vi "Set Speed.vi"(8 "error in (no error)":errorcluster, 10 "Flow Rate (mL/min)":dbl format="%.2f", 11 "VICI Settings In":T1) -> (0 "error out":errorcluster, 1 "Connection Error":bool, 3 "VICI Settings Out":T1)   [LabVIEW 2018, in "VICI M6 M50 Party Mode.lvlib"]
uses:
  VICI M6 M50 Party Mode.lvlib
  Settings Cluster.ctl
  VICI Global Library.lvlib
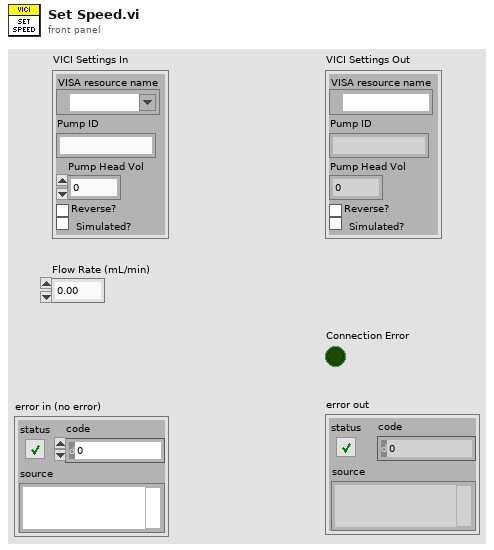
[diagram p1: front panel]
types:
  T1 = typedef "VICI M6 M50 Party Mode.lvlib/Settings Cluster.ctl" = cluster{"VISA resource name":refnum<visa-resource-name>, "Pump ID":string, "Pump Head Vol":dbl, "Reverse?":bool, "Simulated?":bool}
  T2 = typedef "VICI M6 M50 Party Mode.lvlib/VICI Global Library.lvlib/VICI Global.ctl" = cluster{"Busy":bool, "VISA #":string, "Current Pump":string, "Current Function":string, "Pump Array":string[], "Last Success":timestamp, "ID Queue":string[]}
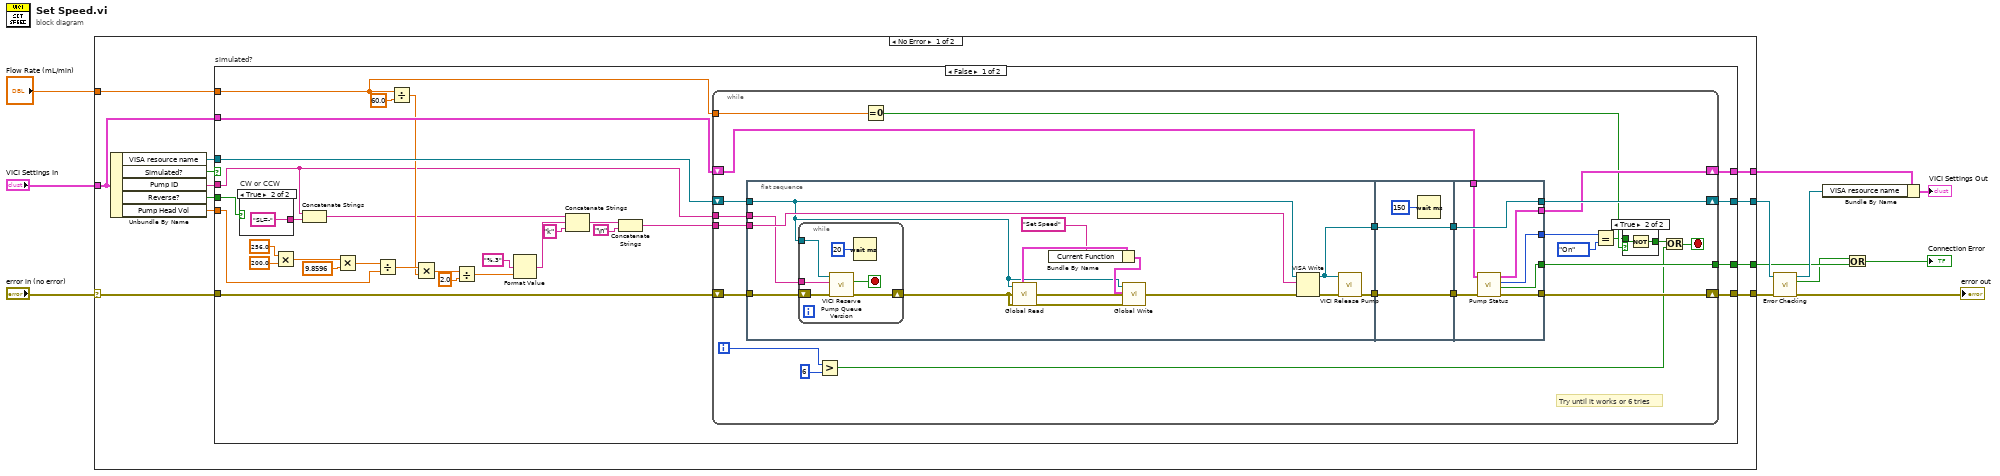
[diagram p0: block diagram]
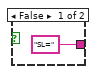
[diagram p3: hidden frame]
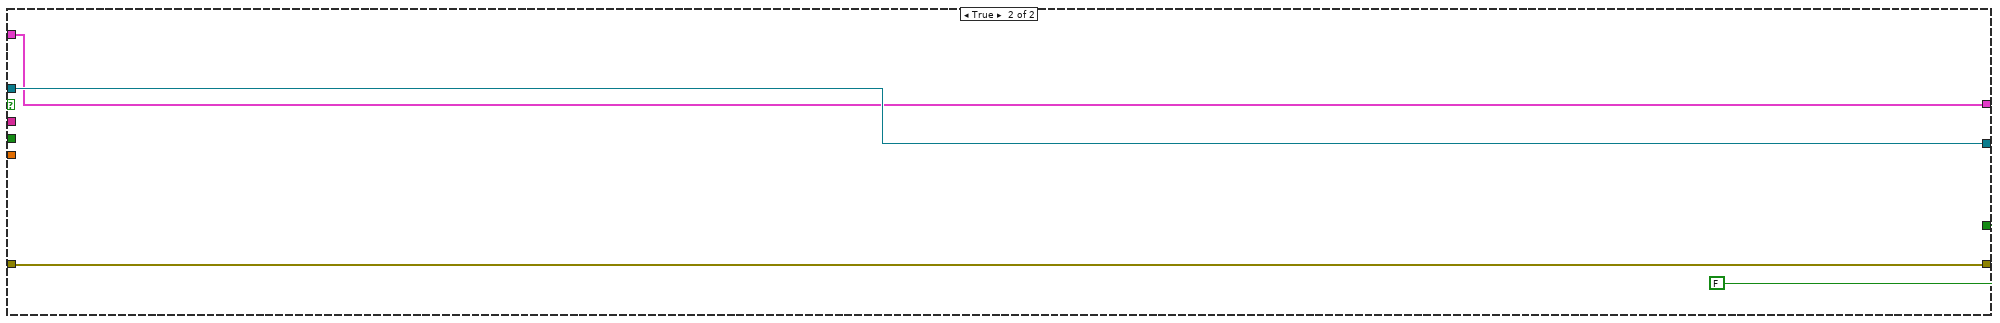
[diagram p4: hidden frame]
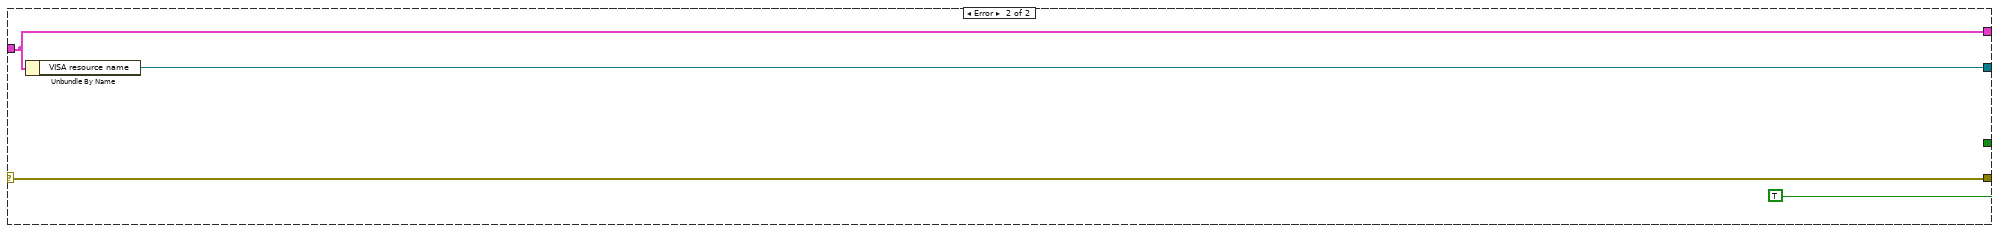
[diagram p5: hidden frame]
diagram:
  n1 = case shown="No Error" "error in (no error)" {
    selector: "error in (no error)" -> [w21 w118]
    tunnel: [w16 w117] -> w6
    tunnel: "VICI Settings In" -> [w17 w117]
    tunnel: "Flow Rate (mL/min)" -> [w20 _]
    tunnel: [w19 w116] -> w10
    tunnel: [w18 w118] -> w9
    tunnel: [w15 TRUE ("Connection Error")] -> w4
    frame No Error {
      n2 = Unbundle By Name(w17) -> ("VISA resource name"=w23:refnum<visa-resource-name>, "Simulated?"=w22:bool, "Pump ID"=w14:string, "Reverse?"=w24:bool, "Pump Head Vol"=w13:dbl)
      n3 = case "simulated?" shown="False" w22 {
        tunnel: [w52 w114] -> w19
        tunnel: w23 -> [w54 w114]
        tunnel: w21 -> [w53 w113]
        tunnel: [w51 w113] -> w18
        tunnel: w24 -> [w50 _]
        tunnel: w20 -> [w29 _]
        tunnel: w17 -> [w49 w112]
        tunnel: [w48 w112] -> w16
        tunnel: [w47 FALSE ("Connection Error")] -> w15
        tunnel: w14 -> [w25 _]
        tunnel: w13 -> [w26 _]
        frame False {
          n4 = case "CW or CCW" shown="True" w50 {
            tunnel: ["SL=" ("string") "SL=-" ("string")] -> w46
            frame False {
            }
            frame True {
            }
          }
          n5 = Multiply(x=256.0, y=200.0) -> (x*y=w31:dbl)
          n6 = Concatenate Strings(w25, w46) -> (w28:string)
          n7 = Multiply(x=w31, y=9.8596) -> (x*y=w41:dbl)
          n8 = Divide(x=w41, y=w26) -> (x/y=w40:dbl)
          n9 = Divide(x=w29, y=60.0) -> (x/y=w39:dbl)
          n10 = Multiply(x=w40, y=w39) -> (x*y=w43:dbl)
          n11 = Divide(x=w43, y=2.0) -> (x/y=w44:dbl)
          n12 = Format Value(format string="%.3", value (0)=w44) -> (output string=w35:string)  [unwired: 1 in]
          n13 = Concatenate Strings(w28, w35, "k" ("string")) -> (w36:string)
          n14 = Concatenate Strings(w36, "\n") -> (w27:string)
          n15 = while {
            shift-right: [w73] -> w52
            shift-left: w54 -> [w65]
            shift-right: [w72] -> w51
            shift-left: w53 -> [w74]
            shift-right: [w70] -> w48
            shift-left: w49 -> [w71]
            tunnel: w29 -> [w69]
            tunnel: [w64] -> w47
            tunnel: w27 -> [w60]
            tunnel: w25 -> [w58]
            i -> [w57]
            stop <- w66 stop-if-true
            # "Try until it works or 6 tries"
            n16 = flat-sequence {
              tunnel: w65 -> [w82]
              tunnel: w74 -> [w89]
              tunnel: [w87] -> w77
              tunnel: w60 -> [w92]
              tunnel: [w90] -> w59
              tunnel: w58 -> [w88]
              tunnel: w77 -> [w101]
              tunnel: [w101] -> w76
              tunnel: [w100] -> w75
              tunnel: w59 -> [w100]
              tunnel: [w106] -> w72
              tunnel: [w108] -> w73
              tunnel: w76 -> [w108]
              tunnel: w75 -> [w107]
              tunnel: w71 -> [w105]
              tunnel: [w104] -> w70
              tunnel: [w103] -> w63
              tunnel: [w102] -> w64
              frame #0 {
                n17 = while {
                  tunnel: w82 -> [w97]
                  tunnel: w88 -> [w96]
                  shift-right: [w93] -> w81
                  shift-left: w89 -> [w95]
                  stop <- w94 stop-if-true
                  n18 = call "VICI Reserve Pump Queue Version.vi"("error in (no error)"=w95, "Pump ID"=w96, "VISA # in"=w97) -> ("error out"=w93:errorcluster, "Loop Completed"=w94:bool)  [unwired: 6 in, 1 out]
                  n19 = Wait (ms)(milliseconds to wait=u32 20) -> ()  [unwired: 1 out]
                }
                n20 = call "Global Read.vi"("VISA #"=w82, "error in (no error)"=w81) -> ("Global for this VISA"=w85:T2, "error out"=w86:errorcluster)  [unwired: 2 in, 5 out]
                n21 = Bundle By Name(cluster=w85, "Current Function"="Set Speed") -> (w84:T2)
                n22 = call "Global Write.vi"("error in (no error)"=w86, "VICI Global"=w84, "VISA # in"=w82) -> ()  [unwired: 7 in, 2 out]
                n23 = VISA Write(VISA resource name=w82, write buffer=w92, error in (no error)=w81) -> (VISA resource name out=w87:refnum<visa-resource-name>, error out=w91:errorcluster)  [unwired: 1 out]
                n24 = call "VICI Release Pump.vi"("error in (no error)"=w91, "VISA # in"=w87) -> ("error out"=w90:errorcluster)  [unwired: 8 in, 1 out]
              }
              frame #1 {
                n25 = Wait (ms)(milliseconds to wait=u32 150) -> ()  [unwired: 1 out]
              }
              frame #2 {
                n26 = call "Pump Status.vi"("error in (no error)"=w107, "VICI Settings In"=w105) -> ("error out"=w106:errorcluster, "Connection Error"=w102:bool, "Pump On?"=w103:enum16{"Off", "On", "Not Initialized"}, "VICI Settings Out"=w104:T1)  [unwired: 6 in]
              }
            }
            n27 = Greater?(x=w57, y=6) -> (0:w56:bool)
            n28 = Equal To 0?(x=w69) -> (x = 0?=w68:bool)
            n29 = Equal?(x=w63, y=enum16{"Off", "On", "Not Initialized"}."On") -> (x = y?=w62:bool)
            n30 = case shown="True" w68 {
              tunnel: [w78 w80] -> w67
              tunnel: w62 -> [w78 w79]
              frame False {
              }
              frame True {
                n31 = Not(x=w79) -> (.not. x?=w80:bool)
              }
            }
            n32 = Or(x=w67, y=w56) -> (x .or. y?=w66:bool)
          }
        }
        frame True {
        }
      }
    }
    frame Error {
      n33 = Unbundle By Name(w117) -> ("VISA resource name"=w116:refnum<visa-resource-name>)
    }
  }
  n34 = call "Error Checking.vi"("error in (no error)"=w9, "VISA resource name"=w10) -> ("error out"=→"error out":errorcluster, "Connection Error"=w3:bool, "VISA resource name"=w7:refnum<visa-resource-name>)  [unwired: 7 in]
  n35 = Bundle By Name(cluster=w6, "VISA resource name"=w7) -> (→"VICI Settings Out":T1)
  n36 = Or(x=w3, y=w4) -> (x .or. y?=→"Connection Error":bool)
